vi "selection_is_dsf.vi"(8 "error in":errorcluster, 11 "vs_tree_control in":refnum<class "vs_tree_control.lvclass">) -> (0 "error out":errorcluster, 2 "is dsf?":bool, 3 "vs_tree_control out":refnum<class "vs_tree_control.lvclass">)   [LabVIEW 2020, in "vs_tree_control.lvclass"]
uses:
  vs_tree_control.lvclass
  vs_tree_control.lvclass/vs_tree_control.ctl
  <vilib>/addons/VeriStand Custom Device Scripting APIs/Data Sharing Framework/Data Sharing Framework Custom Device Scripting.lvlib
  NationalInstruments.VeriStand.SystemStorageUI
  NationalInstruments.VeriStand.SystemStorage
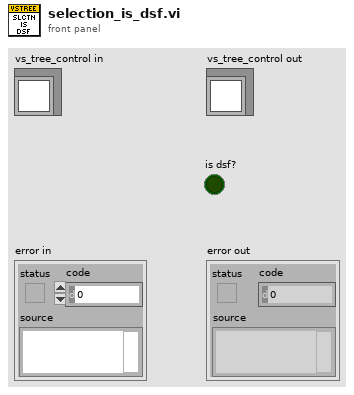
[diagram p1: front panel]
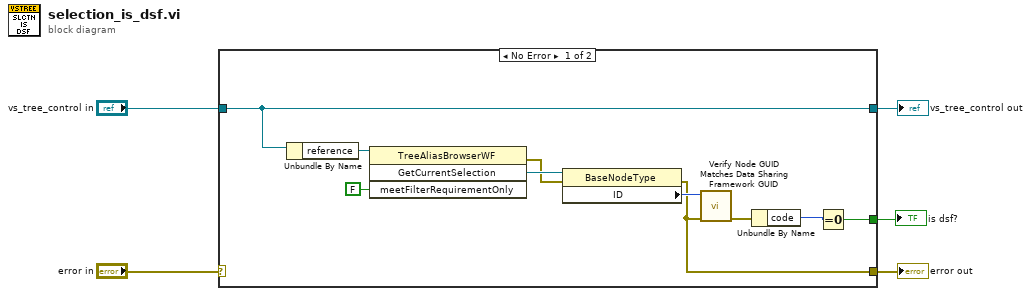
[diagram p0: block diagram]
diagram:
  n1 = case shown="No Error" "error in" {
    selector: "error in" -> [_ w17]
    tunnel: [w7 w17] -> w4
    tunnel: [w11 w16] -> w2
    tunnel: "vs_tree_control in" -> [w11 w16]
    tunnel: [w8 _] -> w1
    frame No Error {
      n2 = Unbundle By Name(w11) -> ("reference"=w10:refnum<k24>)
      n3 = invoke class="TreeAliasBrowserWF" method="GetCurrentSelection"(reference=w10, "meetFilterRequirementOnly"=FALSE) -> (error out=w12:errorcluster, "GetCurrentSelection"=w15:refnum<k24>)  [unwired: 2 in, 2 out]
      n4 = property class="BaseNodeType"(reference=w15, error in=w12) -> (error out=w7:errorcluster, "ID"=w14:u64)  [unwired: 1 out]
      n5 = call <vilib>:"Verify Node GUID Matches Data Sharing Framework GUID.vi"("error in"=w7, "data sharing framework custom device in"=w14) -> ("error out"=w13:errorcluster)  [unwired: 8 in, 1 out]
      n6 = Unbundle By Name(w13) -> ("code"=w9:i32)
      n7 = Equal To 0?(x=w9) -> (x = 0?=w8:bool)
    }
    frame Error {
    }
  }
  "error out" <- w4
  "vs_tree_control out" <- w2
  "is dsf?" <- w1
